vi "BurstInput.vi"(4 "FPGA VI Reference In":refnum<k20>) -> (0 "error out":errorcluster, 1 "Data":u32[](array[numeric]))   [LabVIEW 2011]
uses:
  <vilib>/rvi/interface/nirviMethod/nirviMethod.xnode
  FPGA Bitfiles/FPGA3_FPGATarget_fpga8ch-Main_B3F52CC7.lvbitx
  fpga_8ch-Main.vi
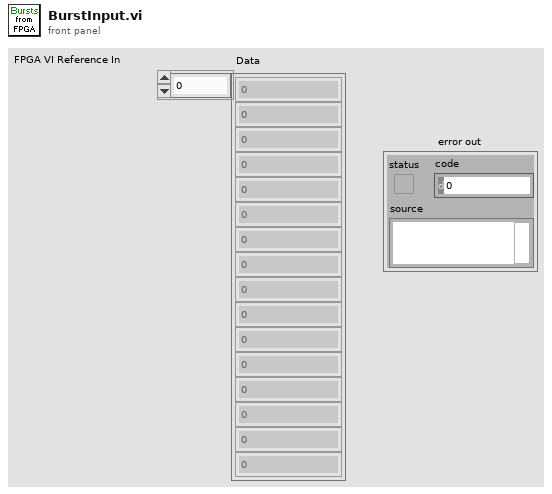
[diagram p1: front panel]
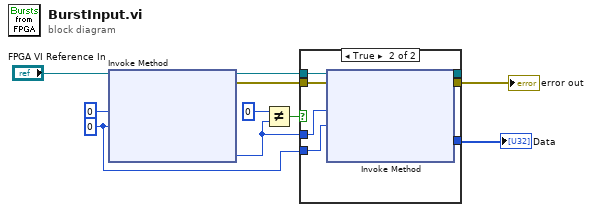
[diagram p0: block diagram]
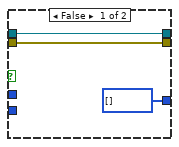
[diagram p2: hidden frame]
diagram:
  w6 = 0 ("Timeout (ms)")
  n1 = xnode "Invoke Method"("FPGA VI Reference In"="FPGA VI Reference In", "Number of Elements"=u32 0, "Timeout (ms)"=w6) -> ("FPGA VI Reference Out"=w5:refnum<k20>, "error out"=w2:errorcluster, "Elements Remaining"=w3:u32)  [unwired: 1 in, 1 out]
  n2 = Not Equal?(x=u32 0 ("y"), y=w3) -> (x != y?=w10:bool)
  n3 = case shown="True" w10 {
    tunnel: w6 -> [_ w16]
    tunnel: [w11 w20] -> _
    tunnel: [w12 w19] -> w9
    tunnel: w3 -> [_ w18]
    tunnel: w5 -> [w11 w17]
    tunnel: w2 -> [w12 w15]
    tunnel: [u32[] [] ("Data") w14] -> w1
    frame False {
    }
    frame True {
      n4 = xnode "Invoke Method"("FPGA VI Reference In"=w17, "error in"=w15, "Number of Elements"=w18, "Timeout (ms)"=w16) -> ("FPGA VI Reference Out"=w20:refnum<k20>, "error out"=w19:errorcluster, "Data"=w14:u32[])  [unwired: 1 out]
    }
  }
  "Data" <- w1
  "error out" <- w9
